vi "MGI Dirty Dot.vi"(7 "Error In":errorcluster, 8 "Cancel? (False)":bool, 9 "Action (Set)":enum16{"Set", "Clear", "Read"}(ring), 10 "VI Reference In (Top Level)":refnum<vi>) -> (0 "Error Out":errorcluster, 2 "Dirty":bool, 3 "VI Reference Out":refnum<vi>)   [LabVIEW 2016]
doc: "Sets, clears, or reads a dirty dot on the Front Panel Title of the referenced VI. \n\nAuthored by Robert C. Mortensen\nsupport@mooregoodideas.com\nwww.mooregoodideas.com\n\nCopyright (c) 2010, Moore Good Ideas, Inc.\n\nAll rights reserved.\n\nRedistribution and use in source and binary forms, with or without modification, are permitted provided that the following conditions are met:\n\n * Redistributions of source code must retain the above copyright notice, this list of conditions and the following disclaimer.\n * Redistributions in binary form must reproduce the above copyright notice, this list of conditions and the following disclaimer in the documentation and/or other materials provided with the distribution.\n * Neither the name of Moore Good Ideas, Inc. nor the names of its contributors may be used to endorse or promote products derived from this software without specific prior written permission.\n\nTHIS SOFTWARE IS PROVIDED BY THE COPYRIGHT HOLDERS AND CONTRIBUTORS \"AS IS\" AND ANY EXPRESS OR IMPLIED WARRANTIES, INCLUDING, BUT NOT LIMITED TO, THE IMPLIED WARRANTIES OF MERCHANTABILITY AND FITNESS FOR A PARTICULAR PURPOSE ARE DISCLAIMED. IN NO EVENT SHALL THE COPYRIGHT OWNER OR CONTRIBUTORS BE LIABLE FOR ANY DIRECT, INDIRECT, INCIDENTAL, SPECIAL, EXEMPLARY, OR CONSEQUENTIAL DAMAGES (INCLUDING, BUT NOT LIMITED TO, PROCUREMENT OF SUBSTITUTE GOODS OR SERVICES; LOSS OF USE, DATA, OR PROFITS; OR BUSINESS INTERRUPTION) HOWEVER CAUSED AND ON ANY THEORY OF LIABILITY, WHETHER IN CONTRACT, STRICT LIABILITY, OR TORT (INCLUDING NEGLIGENCE OR OTHERWISE) ARISING IN ANY WAY OUT OF THE USE OF THIS SOFTWARE, EVEN IF ADVISED OF THE POSSIBILITY OF SUCH DAMAGE."
uses:
  <userlib>/_MGI/Application Control/MGI VI Reference/MGI Top Level VI Reference.vi
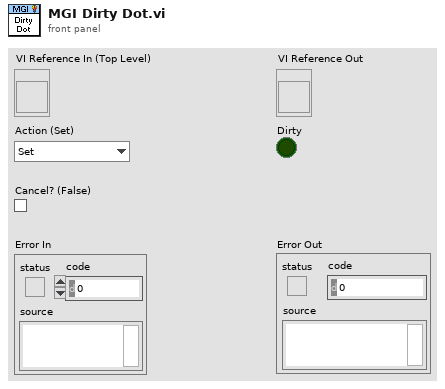
[diagram p1: front panel]
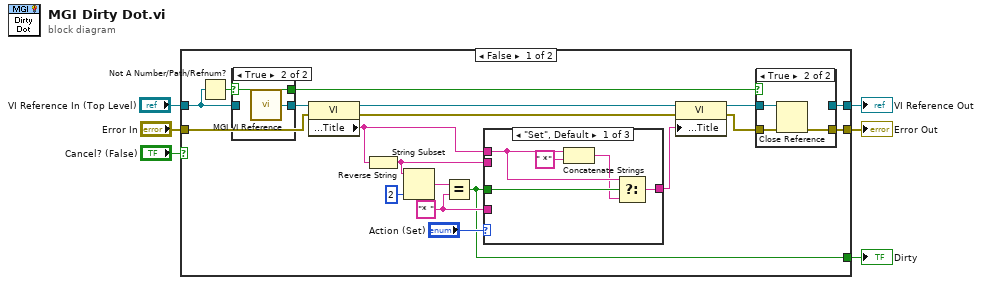
[diagram p0: block diagram]
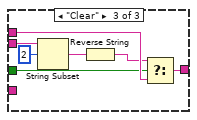
[diagram p5: hidden frame]
diagram:
  n1 = case shown="False" "Cancel? (False)" {
    tunnel: [w12 w48] -> w6
    tunnel: [w15 _] -> w4
    tunnel: "Error In" -> [w8 w48]
    tunnel: "VI Reference In (Top Level)" -> [w10 w47]
    tunnel: [w7 w47] -> w1
    frame False {
      w18 = "* " ("y")
      n2 = Not A Number/Path/Refnum?(number/path/refnum=w10) -> (NaN/Path/Refnum?=w11:bool)
      n3 = case shown="True" w11 {
        selector: w11 -> [_ w33]
        tunnel: [w31 w32] -> w25
        tunnel: w10 -> [w31 _]
        tunnel: [_ w33] -> w9
        frame False {
        }
        frame True {
          n4 = call-poly <userlib>:"MGI VI Reference.vi"() -> ("Top Level VI Reference"=w32:refnum<vi>)  [unwired: 1 in]
        }
      }
      n5 = property class="VI"(reference=w25, error in=w8) -> (reference out=w24:refnum<vi>, error out=w23:errorcluster, "Front Panel Window:Title"=w20:string)
      n6 = Reverse String(1:w20) -> (0:w16:string)
      n7 = String Subset(string=w16, length (rest)=2 ("length (rest)")) -> (substring=w19:string)  [unwired: 1 in]
      n8 = Equal?(x=w19, y=w18) -> (x = y?=w15:bool)
      n9 = case shown="\"Set\", Default" "Action (Set)" {
        tunnel: w20 -> [w37 w39 w45]
        tunnel: w15 -> [w38 _ w40]
        tunnel: w18 -> [_ _ _]
        tunnel: [w36 w39 w46] -> w17
        tunnel: w16 -> [_ _ w44]
        frame "Set", Default {
          n10 = Concatenate Strings(w37, " *" ("string")) -> (w35:string)
          n11 = Select(t=w37, s=w38, f=w35) -> (s? t:f=w36:string)
        }
        frame "Read" {
        }
        frame "Clear" {
          n12 = String Subset(string=w44, offset (0)=2) -> (substring=w41:string)  [unwired: 1 in]
          n13 = Reverse String(1:w41) -> (0:w42:string)
          n14 = Select(t=w42, s=w40, f=w45) -> (s? t:f=w46:string)
        }
      }
      n15 = property class="VI"(reference=w24, error in=w23, "Front Panel Window:Title"=w17) -> (reference out=w14:refnum<vi>, error out=w13:errorcluster)
      n16 = case shown="True" w9 {
        tunnel: w14 -> [w26 w30]
        tunnel: w13 -> [w27 w29]
        tunnel: [w27 w28] -> w12
        tunnel: [w26 _] -> w7
        frame False {
        }
        frame True {
          n17 = Close Reference(reference=w30, error in (no error)=w29) -> (error out=w28:errorcluster)
        }
      }
    }
    frame True {
    }
  }
  "Error Out" <- w6
  "Dirty" <- w4
  "VI Reference Out" <- w1
